vi "submain.vi"   [LabVIEW 2019]
uses:
  Global Variables/global.vi
  Global Variables/Data_Display_global.vi
  Instrument_Setup.vi
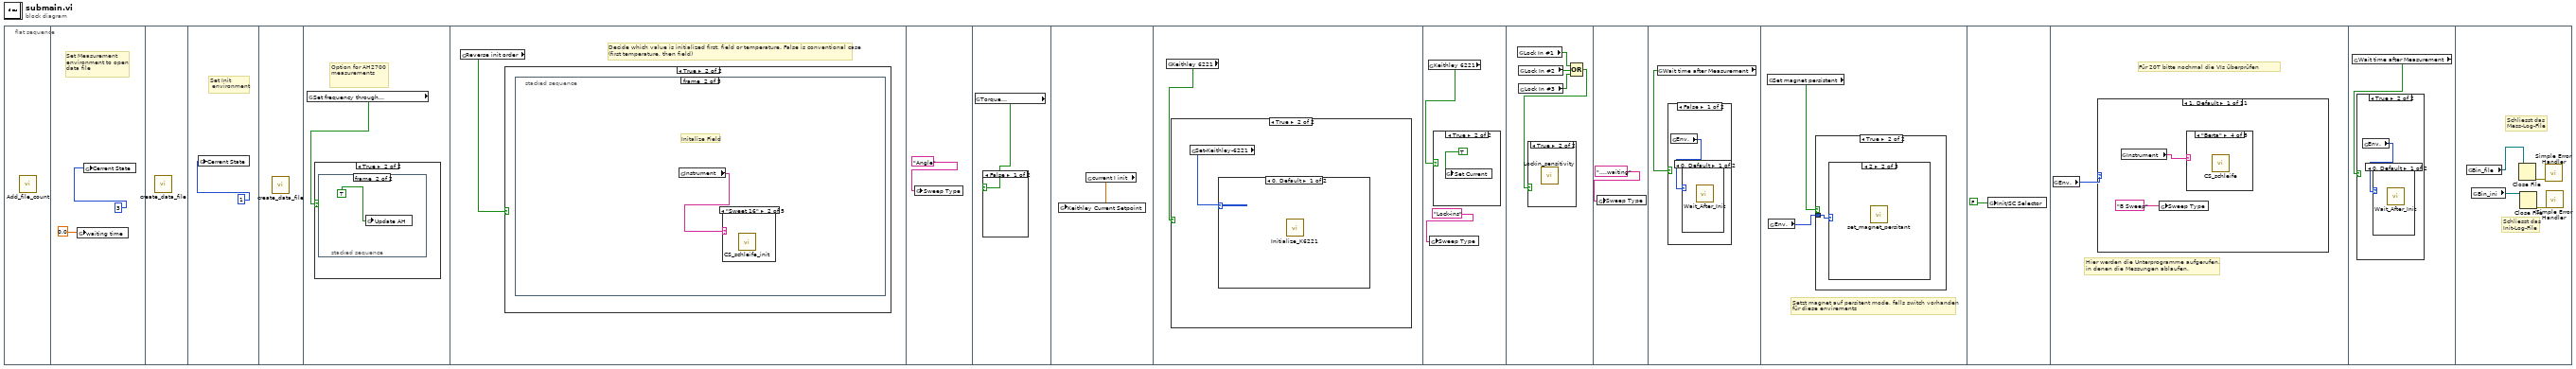
[diagram p0: block diagram]
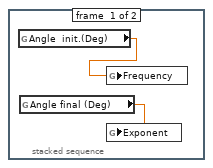
[diagram p3: hidden frame]
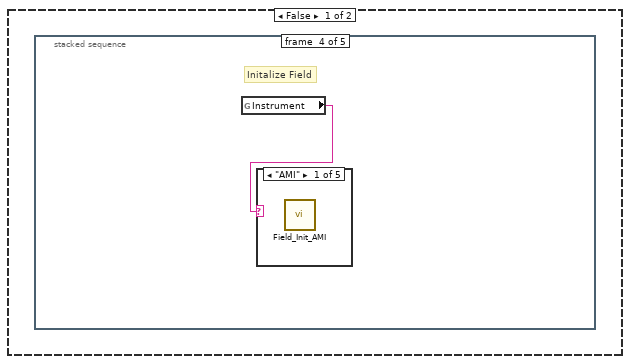
[diagram p4: hidden frame]
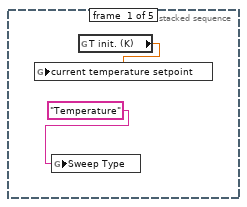
[diagram p5: hidden frame]
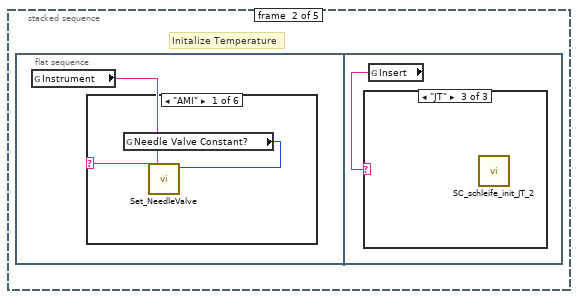
[diagram p6: hidden frame]
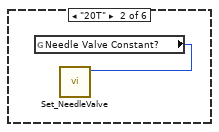
[diagram p7: hidden frame]
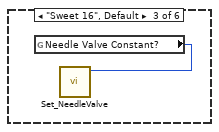
[diagram p8: hidden frame]
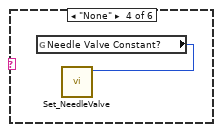
[diagram p9: hidden frame]
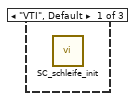
[diagram p12: hidden frame]
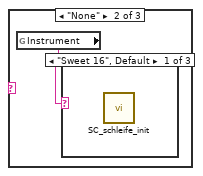
[diagram p13: hidden frame]
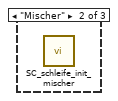
[diagram p14: hidden frame]
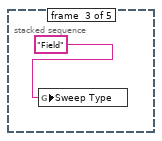
[diagram p16: hidden frame]
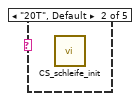
[diagram p17: hidden frame]
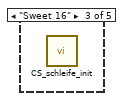
[diagram p18: hidden frame]
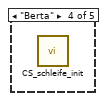
[diagram p19: hidden frame]
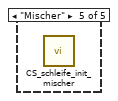
[diagram p20: hidden frame]
diagram:
  n1 = flat-sequence {
    frame #0 {
      n2 = call "Add_file_count.vi"() -> ()  [unwired: 12 in]
    }
    frame #1 {
      # "Set Measurement\nenvironment to open\ndata file"
      n3 = global write "Data_Display_global.vi" "waiting time"(0.0) -> ()
      n4 = global write "global.vi" "Cerrent State"(3) -> ()
    }
    frame #2 {
      n5 = call "create_data_file.vi"() -> ()  [unwired: 3 in]
    }
    frame #3 {
      # "Set Init\n environment"
      n6 = global write "global.vi" "Cerrent State"(1) -> ()
    }
    frame #4 {
      n7 = call "create_data_file.vi"() -> ()  [unwired: 3 in]
    }
    frame #5 {
      # "Option for AH2700 \nmeasurements"
      n8 = global read "Instrument_Setup.vi" "Set frequency through\ncommand file"() -> (w4:bool)
      n9 = case shown="True" w4 {
        frame False {
        }
        frame True {
          n10 = stacked-sequence {
            frame #0 {
              n11 = global read "global.vi" "Angle  init.(Deg)"() -> (w6:dbl)
              n12 = global read "global.vi" "Angle final (Deg)"() -> (w5:dbl)
              n13 = global write "global.vi" "Frequency"(w6) -> ()
              n14 = global write "global.vi" "Exponent"(w5) -> ()
            }
            frame #1 {
              n15 = global write "Data_Display_global.vi" "Update AH"(TRUE) -> ()
            }
          }
        }
      }
    }
    frame #6 {
      # "Decide which value is initialized first, field or temperature. False is conventional case\n(first temperature, then field)"
      n16 = global read "Instrument_Setup.vi" "Reverse init order"() -> (w8:bool)
      n17 = case shown="True" w8 {
        frame False {
          n18 = stacked-sequence {
            frame #0 {
              n19 = global write "global.vi" "Sweep Type"("Temperature") -> ()
              n20 = global read "global.vi" "T init. (K)"() -> (w9:dbl)
              n21 = global write "Data_Display_global.vi" "current temperature setpoint"(w9) -> ()
            }
            frame #1 {
              # "Initalize Temperature"
              n22 = flat-sequence {
                frame #0 {
                  n23 = global read "Instrument_Setup.vi" "Instrument"() -> (w11:string)
                  n24 = case shown="\"AMI\"" w11 {
                    frame "AMI" {
                      n25 = global read "global.vi" "Needle Valve Constant?"() -> (w12:i32)
                      n26 = call "Set_NeedleValve.vi"("Numeric"=w12) -> ()  [unwired: 11 in]
                    }
                    frame "20T" {
                      n27 = global read "global.vi" "Needle Valve Constant?"() -> (w13:i32)
                      n28 = call "Set_NeedleValve.vi"("Numeric"=w13) -> ()  [unwired: 11 in]
                    }
                    frame "Sweet 16", Default {
                      n29 = global read "global.vi" "Needle Valve Constant?"() -> (w14:i32)
                      n30 = call "Set_NeedleValve.vi"("Numeric"=w14) -> ()  [unwired: 11 in]
                    }
                    frame "None" {
                      n31 = global read "global.vi" "Needle Valve Constant?"() -> (w15:i32)
                      n32 = call "Set_NeedleValve.vi"("Numeric"=w15) -> ()  [unwired: 11 in]
                    }
                    frame "Mischer" {
                    }
                    frame "Berta" {
                    }
                  }
                }
                frame #1 {
                  n33 = global read "Instrument_Setup.vi" "Insert"() -> (w16:string)
                  n34 = case shown="\"JT\"" w16 {
                    frame "VTI", Default {
                      n35 = call "SC_schleife_init.vi"() -> ()  [unwired: 4 in]
                    }
                    frame "None" {
                      n36 = global read "Instrument_Setup.vi" "Instrument"() -> (w17:string)
                      n37 = case shown="\"Sweet 16\", Default" w17 {
                        frame "Sweet 16", Default {
                          n38 = call "SC_schleife_init.vi"() -> ()  [unwired: 4 in]
                        }
                        frame "Mischer" {
                          n39 = call "SC_schleife_init_mischer.vi"() -> ()  [unwired: 4 in]
                        }
                        frame "Berta" {
                        }
                      }
                    }
                    frame "JT" {
                      n40 = call "SC_schleife_init_JT_2.vi"() -> ()  [unwired: 4 in]
                    }
                  }
                }
              }
            }
            frame #2 {
              n41 = global write "global.vi" "Sweep Type"("Field") -> ()
            }
            frame #3 {
              # "Initalize Field"
              n42 = global read "Instrument_Setup.vi" "Instrument"() -> (w19:string)
              n43 = case shown="\"AMI\"" w19 {
                frame "AMI" {
                  n44 = call "Field_Init_AMI.vi"() -> ()  [unwired: 3 in]
                }
                frame "20T", Default {
                  n45 = call "CS_schleife_init.vi"() -> ()  [unwired: 4 in]
                }
                frame "Sweet 16" {
                  n46 = call "CS_schleife_init.vi"() -> ()  [unwired: 4 in]
                }
                frame "Berta" {
                  n47 = call "CS_schleife_init.vi"() -> ()  [unwired: 4 in]
                }
                frame "Mischer" {
                  n48 = call "CS_schleife_init_mischer.vi"() -> ()  [unwired: 4 in]
                }
              }
            }
            frame #4 {
              # "Set field persistent"
              n49 = global read "global.vi" "Env."() -> (w20:i32)
              n50 = case shown="0, Default" w20 {
                frame 0, Default {
                  n51 = global read "Instrument_Setup.vi" "Instrument"() -> (w21:string)
                  n52 = case shown="\"AMI\"" w21 {
                    frame "20T", Default {
                      n53 = call "Set_Persistent.vi"() -> ()  [unwired: 12 in]
                    }
                    frame "AMI" {
                      n54 = call "Set_Persistent.vi"() -> ()  [unwired: 12 in]
                    }
                    frame "Mischer" {
                    }
                    frame "Berta" {
                      n55 = call "Set_Persistent.vi"() -> ()  [unwired: 12 in]
                    }
                    frame "Sweet 16" {
                      n56 = call "Set_Persistent.vi"() -> ()  [unwired: 12 in]
                    }
                  }
                }
                frame 1 {
                }
                frame 4 {
                }
              }
            }
          }
        }
        frame True {
          n57 = stacked-sequence {
            frame #0 {
              n58 = global write "global.vi" "Sweep Type"("Field") -> ()
            }
            frame #1 {
              # "Initalize Field"
              n59 = global read "Instrument_Setup.vi" "Instrument"() -> (w23:string)
              n60 = case shown="\"Sweet 16\"" w23 {
                frame "AMI" {
                  n61 = call "Field_Init_AMI.vi"() -> ()  [unwired: 3 in]
                }
                frame "Sweet 16" {
                  n62 = call "CS_schleife_init.vi"() -> ()  [unwired: 4 in]
                }
                frame "Mischer" {
                  n63 = call "CS_schleife_init_mischer.vi"() -> ()  [unwired: 4 in]
                }
                frame "20T", Default {
                }
                frame "Berta" {
                  n64 = call "CS_schleife_init.vi"() -> ()  [unwired: 4 in]
                }
              }
            }
            frame #2 {
              n65 = global read "global.vi" "Env."() -> (w24:i32)
              n66 = case shown="0, Default" w24 {
                frame 0, Default {
                  n67 = global read "Instrument_Setup.vi" "Instrument"() -> (w25:string)
                  n68 = case shown="\"AMI\"" w25 {
                    frame "20T", Default {
                      n69 = call "Set_Persistent.vi"() -> ()  [unwired: 12 in]
                    }
                    frame "AMI" {
                      n70 = call "Set_Persistent.vi"() -> ()  [unwired: 12 in]
                    }
                    frame "Mischer" {
                    }
                    frame "Berta" {
                      n71 = call "Set_Persistent.vi"() -> ()  [unwired: 12 in]
                    }
                    frame "Sweet 16" {
                      n72 = call "Set_Persistent.vi"() -> ()  [unwired: 12 in]
                    }
                  }
                }
                frame 1 {
                }
                frame 4 {
                }
              }
            }
            frame #3 {
              n73 = global read "global.vi" "T init. (K)"() -> (w26:dbl)
              n74 = global write "Data_Display_global.vi" "current temperature setpoint"(w26) -> ()
              n75 = global write "global.vi" "Sweep Type"("Temperature") -> ()
            }
            frame #4 {
              # "Initalize Temperature"
              n76 = flat-sequence {
                frame #0 {
                  n77 = global read "Instrument_Setup.vi" "Insert"() -> (w28:string)
                  n78 = case shown="\"VTI\", Default" w28 {
                    frame "JT" {
                    }
                    frame "VTI", Default {
                      n79 = global read "global.vi" "Needle Valve Constant?"() -> (w29:i32)
                      n80 = call "Set_NeedleValve.vi"("Numeric"=w29) -> ()  [unwired: 11 in]
                    }
                    frame "20TVTI" {
                    }
                    frame "None" {
                    }
                  }
                }
                frame #1 {
                  n81 = global read "Instrument_Setup.vi" "T-control"() -> (w30:string)
                  n82 = case shown="\"Insert-control\", Default" w30 {
                    frame "LS372" {
                      n83 = call "SC_schleife_init_mischer.vi"() -> ()  [unwired: 4 in]
                    }
                    frame "LS370" {
                      n84 = call "SC_schleife_init_JT_2.vi"() -> ()  [unwired: 4 in]
                    }
                    frame "None" {
                    }
                    frame "Insert-control", Default {
                      n85 = global read "Instrument_Setup.vi" "Insert"() -> (w31:string)
                      n86 = case shown="\"JT\"" w31 {
                        frame "VTI", Default {
                          n87 = call "SC_schleife_init.vi"() -> ()  [unwired: 4 in]
                        }
                        frame "None" {
                        }
                        frame "20TVTI" {
                        }
                        frame "JT" {
                          n88 = call "SC_schleife_init_JT_2.vi"() -> ()  [unwired: 4 in]
                        }
                      }
                    }
                  }
                }
              }
            }
          }
        }
      }
    }
    frame #7 {
      n89 = global write "global.vi" "Sweep Type"("Angle") -> ()
    }
    frame #8 {
      n90 = global read "Instrument_Setup.vi" "Torque \nMeasurem."() -> (w33:bool)
      n91 = case shown="False" w33 {
        frame False {
        }
        frame True {
          n92 = call "Angle_init.vi"() -> ()  [unwired: 12 in]
        }
      }
    }
    frame #9 {
      n93 = global read "global.vi" "current I init"() -> (w34:dbl)
      n94 = global write "Data_Display_global.vi" "Keithley Current Setpoint"(w34) -> ()
    }
    frame #10 {
      n95 = global read "Instrument_Setup.vi" "Keithley 6221"() -> (w35:bool)
      n96 = case shown="True" w35 {
        frame False {
        }
        frame True {
          n97 = global read "Instrument_Setup.vi" "Set-Keithley-6221"() -> (w36:u16)
          n98 = case shown="0, Default" w36 {
            frame 0, Default {
              n99 = call "Initialize_K6221.vi"() -> ()  [unwired: 12 in]
            }
            frame 1 {
            }
          }
        }
      }
    }
    frame #11 {
      n100 = global read "Instrument_Setup.vi" "Keithley 6221"() -> (w37:bool)
      n101 = global write "global.vi" "Sweep Type"("Lock-ins") -> ()
      n102 = case shown="True" w37 {
        frame False {
        }
        frame True {
          n103 = global write "Data_Display_global.vi" "Set Current"(TRUE) -> ()
        }
      }
    }
    frame #12 {
      n104 = global read "Instrument_Setup.vi" "Lock In #1"() -> (w43:bool)
      n105 = global read "Instrument_Setup.vi" "Lock In #2"() -> (w42:bool)
      n106 = global read "Instrument_Setup.vi" "Lock In #3"() -> (w41:bool)
      n107 = Compound Arithmetic op=OR(w43, w42, w41) -> (w40:bool)
      n108 = case shown="True" w40 {
        frame False {
        }
        frame True {
          n109 = call "Lockin_sensitivity.vi"() -> ()  [unwired: 12 in]
        }
      }
    }
    frame #13 {
      n110 = global write "global.vi" "Sweep Type"("....waiting") -> ()
    }
    frame #14 {
      n111 = global read "Instrument_Setup.vi" "Wait time after Measurement"() -> (w45:bool)
      n112 = case shown="False" w45 {
        frame False {
          n113 = global read "global.vi" "Env."() -> (w46:i32)
          n114 = case shown="0, Default" w46 {
            frame 0, Default {
              n115 = call "Wait_After_Init.vi"() -> ()  [unwired: 12 in]
            }
            frame 3 {
            }
          }
        }
        frame True {
        }
      }
    }
    frame #15 {
      # "Setzt magnet auf persitent mode, falls switch vorhanden\nfür diese envirements"
      n116 = global read "Instrument_Setup.vi" "Set magnet persistent"() -> (w48:bool)
      n117 = global read "global.vi" "Env."() -> (w47:i32)
      n118 = case shown="True" w48 {
        tunnel: w47 -> [_ w49]
        frame False {
        }
        frame True {
          n119 = case shown="2" w49 {
            frame 1, Default {
            }
            frame 2 {
              n120 = call "set_magnet_persitant.vi"() -> ()  [unwired: 4 in]
            }
            frame 10 {
              n121 = call "set_magnet_persitant.vi"() -> ()  [unwired: 4 in]
            }
          }
        }
      }
    }
    frame #16 {
      n122 = global write "Data_Display_global.vi" "Init/SC Selector"(FALSE ("Init/SC Selector")) -> ()
    }
    frame #17 {
      # "Für 20T bitte nochmal die VIs überprüfen"
      # "Hier werden die Unterprogramme aufgerufen,\nin denen die Messungen ablaufen."
      n123 = global read "global.vi" "Env."() -> (w51:i32)
      n124 = case shown="1, Default" w51 {
        frame 1, Default {
          n125 = global read "Instrument_Setup.vi" "Instrument"() -> (w52:string)
          n126 = global write "global.vi" "Sweep Type"("B Sweep") -> ()
          n127 = case shown="\"Berta\"" w52 {
            frame "AMI" {
              n128 = call "Field_Sweep_AMI.vi"() -> ()  [unwired: 3 in]
            }
            frame "20T", Default {
              n129 = call "CS_schleife.vi"() -> ()  [unwired: 4 in]
            }
            frame "Sweet 16" {
              n130 = call "CS_schleife.vi"() -> ()  [unwired: 4 in]
            }
            frame "Berta" {
              n131 = call "CS_schleife.vi"() -> ()  [unwired: 4 in]
            }
            frame "Mischer" {
              n132 = call "CS_schleife.vi"() -> ()  [unwired: 4 in]
            }
          }
        }
        frame 2 {
          # "Temperature Sweep"
          n133 = global read "Instrument_Setup.vi" "T-control"() -> (w54:string)
          n134 = case shown="\"Insert-control\", Default" w54 {
            frame "None" {
            }
            frame "LS370" {
              n135 = call "SC_schleife_JT.vi"() -> ()  [unwired: 4 in]
            }
            frame "LS372" {
              n136 = call "SC_schleife_mischer.vi"() -> ()  [unwired: 4 in]
            }
            frame "Insert-control", Default {
              n137 = global read "Instrument_Setup.vi" "Insert"() -> (w56:string)
              n138 = case shown="\"VTI\", Default" w56 {
                frame "VTI", Default {
                  n139 = call "SC_schleife.vi"() -> ()  [unwired: 4 in]
                }
                frame "20TVTI" {
                }
                frame "JT" {
                  n140 = call "SC_schleife_JT.vi"() -> ()  [unwired: 4 in]
                }
                frame "None" {
                }
              }
            }
          }
          n141 = global write "global.vi" "Sweep Type"("T Sweep") -> ()
        }
        frame 3 {
          n142 = stacked-sequence {
            frame #0 {
              n143 = global write "global.vi" "Cerrent State"(4) -> ()
            }
            frame #1 {
              n144 = call "Const_loop.vi"() -> ()  [unwired: 4 in]
              n145 = global write "global.vi" "Sweep Type"("Const") -> ()
            }
          }
        }
        frame 4 {
          # "Feld Step"
          n146 = global read "Instrument_Setup.vi" "Instrument"() -> (w59:string)
          n147 = global write "global.vi" "Sweep Type"("B Step") -> ()
          n148 = case shown="\"AMI\"" w59 {
            frame "Sweet 16", Default {
            }
            frame "AMI" {
              n149 = call "Field_Step_AMI.vi"() -> ()  [unwired: 3 in]
            }
          }
        }
        frame 5 {
          # "Current Step"
          n150 = global write "global.vi" "Sweep Type"("I Step") -> ()
          n151 = call "Current_Step.vi"() -> ()  [unwired: 1 in]
        }
        frame 6 {
          # "Temperature Step"
          n152 = global read "Instrument_Setup.vi" "T-control"() -> (w62:string)
          n153 = case shown="\"Insert-control\"" w62 {
            frame "None", Default {
            }
            frame "LS370" {
              n154 = call "T_step_JT.vi"() -> ()  [unwired: 3 in]
            }
            frame "LS372" {
              n155 = call "T_step_mischer.vi"() -> ()  [unwired: 3 in]
            }
            frame "Insert-control" {
              n156 = global read "Instrument_Setup.vi" "Insert"() -> (w64:string)
              n157 = case shown="\"JT\", Default" w64 {
                frame "VTI" {
                  n158 = call "T_step_VTI.vi"() -> ()  [unwired: 3 in]
                }
                frame "JT", Default {
                  n159 = call "T_step_JT.vi"() -> ()  [unwired: 3 in]
                }
                frame "20TVTI" {
                }
                frame "None" {
                }
              }
            }
          }
          n160 = global write "global.vi" "Sweep Type"("T Step") -> ()
        }
        frame 7 {
          n161 = call "Angle_Step.vi"() -> ()  [unwired: 3 in]
          n162 = global write "global.vi" "Sweep Type"("Angle Step") -> ()
        }
        frame 8 {
          n163 = global write "global.vi" "Sweep Type"("Freq Step") -> ()
          n164 = call "Frequ-sweep.vi"() -> ()  [unwired: 4 in]
        }
        frame 10 {
          n165 = global write "global.vi" "Sweep Type"("Amp Step") -> ()
          n166 = call "Amp-sweep.vi"() -> ()  [unwired: 4 in]
        }
        frame 9 {
          n167 = global write "global.vi" "Sweep Type"("Calibration") -> ()
          n168 = call "Calibration_AH2700.vi"() -> ()  [unwired: 18 in, 2 out]
        }
        frame 11 {
          n169 = global write "global.vi" "Sweep Type"("Field and T scan") -> ()
          n170 = call "Field_and_Temperature_sweep_at the same _time.vi"() -> ()  [unwired: 12 in]
        }
      }
    }
    frame #18 {
      n171 = global read "Instrument_Setup.vi" "Wait time after Measurement"() -> (w70:bool)
      n172 = case shown="True" w70 {
        frame False {
        }
        frame True {
          n173 = global read "global.vi" "Env."() -> (w71:i32)
          n174 = case shown="0, Default" w71 {
            frame 0, Default {
              n175 = call "Wait_After_Init.vi"() -> ()  [unwired: 12 in]
            }
            frame 3 {
            }
          }
        }
      }
    }
    frame #19 {
      # "Schliesst das\nInit-Log-File"
      # "Schliesst das\nMess-Log-File"
      n176 = global read "Instrument_Setup.vi" "Bin_file"() -> (w73:refnum<file>)
      n177 = global read "Instrument_Setup.vi" "Bin_ini"() -> (w72:refnum<file>)
      n178 = Close File(refnum=w73) -> (error out=w74:errorcluster)  [unwired: 1 in, 1 out]
      n179 = Close File(refnum=w72) -> (error out=w75:errorcluster)  [unwired: 1 in, 1 out]
      n180 = call <vilib>:"Simple Error Handler.vi"("error in (no error)"=w74) -> ()  [unwired: 4 in, 5 out]
      n181 = call <vilib>:"Simple Error Handler.vi"("error in (no error)"=w75) -> ()  [unwired: 4 in, 5 out]
    }
  }
